vi "seno_gradino.vi"(0 "ampiezza [V]":dbl=10.0, 1 "scelta_funzione":bool, 2 "Gradino_AMP?":bool, 3 "Gradino_FASE?":bool, 5 "frequenza[Hz]":dbl=50.0, 7 "Variazione Percentuale [%]":dbl, 9 "fase[°]":dbl, 11 "Gradi innalzamento[°]":dbl, 12 "rate [sample/s]":dbl=10000.0, 13 "t0[s]":dbl, 14 "lunghezza finestra[s]":dbl=0.06) -> (4 "Waveform Graph":dbl[](graph)=[6.123233995736766e-16, -0.3141075907812828, -0.627905195293134, -0.9410831331851417, -1.2533323356430415, -1.5643446504023082, -1.873813145857246, -2.1814324139654255, -2.4868988716485463, -2.7899110603922934, -3.0901699437494736, -3.3873792024529137, -3.6812455268467796, -3.971478906347807, -4.257792915650727, -4.539904997395467, -4.81753674101715, -5.090414157503713, -5.358267949789969, -5.620833778521307, -5.87785252292473, -6.129070536529766, -6.3742398974868975, -6.613118653236517, -6.845471059286887, -7.071067811865475, -7.289686274214117, -7.501110696304596, -7.705132427757891, -7.901550123756904, -8.090169943749473, -8.270805742745619, -8.443279255020151, -8.607420270039437, -8.763066800438637, -8.910065241883679, -9.048270524660197, -9.177546256839811, -9.297764858882514, -9.408807689542254, -9.510565162951535, -9.60293685676943, -9.685831611286313, -9.759167619387474, -9.822872507286887, -9.876883405951377, -9.921147013144777, -9.9556196460308, -9.980267284282716, -9.995065603657316, -10.0, -9.995065603657316, -9.980267284282716, -9.9556196460308, -9.921147013144779, -9.876883405951379, -9.822872507286887, -9.759167619387474, -9.68583161128631, -9.60293685676943, -9.510565162951536, -9.408807689542254, -9.297764858882513, -9.177546256839811, -9.048270524660195, -8.910065241883677, -8.763066800438635, -8.607420270039437, -8.44327925502015, -8.270805742745619, -8.090169943749476, -7.901550123756903, -7.70513242775789, -7.501110696304597, -7.289686274214116, -7.071067811865474, -6.845471059286886, -6.613118653236519, -6.374239897486895, -6.129070536529765, -5.877852522924733, -5.620833778521309, -5.358267949789964, -5.0904141575037105, -4.817536741017145, -4.539904997395461, -4.257792915650722, -3.971478906347803, -3.6812455268467783, -3.3873792024529137, -3.0901699437494754, -2.789911060392296, -2.486898871648553, -2.1814324139654238, -1.8738131458572462, -1.5643446504023104, -1.2533323356430373, -0.9410831331851397, -0.627905195293132, -0.314107590781283, -1.8369701987210296e-15, 0.3141075907812882, 0.6279051952931372, 0.9410831331851449, 1.2533323356430512, 1.5643446504023157, 1.8738131458572513, 2.181432413965429, 2.4868988716485494, 2.789911060392292, 3.0901699437494723, 3.3873792024529106, 3.6812455268467743, 3.9714789063478073, 4.257792915650726, 4.539904997395467, 4.8175367410171575, 5.090414157503716, 5.358267949789967, 5.620833778521305, 5.877852522924729, 6.1290705365297695, 6.3742398974869, 6.613118653236519, 6.845471059286893, 7.07106781186548, 7.289686274214119, 7.501110696304597, 7.705132427757894, 7.901550123756903, 8.090169943749478, 8.27080574274562, 8.443279255020153, 8.607420270039437, 8.763066800438637, 8.910065241883679, 9.048270524660197, 9.177546256839813, 9.297764858882514, 9.408807689542254, 9.510565162951535, 9.602936856769432, 9.685831611286313, 9.759167619387474, 9.822872507286888, 9.876883405951377, 9.921147013144777, 9.9556196460308, 9.980267284282716, 9.995065603657316, 10.0, 9.995065603657315, 9.980267284282716, 9.9556196460308, 9.921147013144779, 9.876883405951379, 9.822872507286887, 9.759167619387473, 9.68583161128631, 9.60293685676943, 9.510565162951536, 9.408807689542256, 9.297764858882516, 9.177546256839808, 9.048270524660191, 8.910065241883675, 8.763066800438633, 8.607420270039436, 8.443279255020146, 8.270805742745614, 8.09016994374947, 7.901550123756901, 7.70513242775789, 7.501110696304595, 7.28968627421411, 7.071067811865471, 6.845471059286884, 6.613118653236517, 6.374239897486897, 6.129070536529766, 5.8778525229247265, 5.620833778521303, 5.358267949789965, 5.090414157503712, 4.817536741017154, 4.539904997395462, 4.257792915650723, 3.971478906347804, 3.681245526846779, 3.387379202452915, 3.090169943749477, 2.7899110603922885, 2.486898871648546, 2.181432413965425, 1.8738131458572473, 1.5643446504023117, 1.2533323356430472, 0.941083133185132, 0.6279051952931332, 0.31410759078128425, 3.061616997868383e-15, -0.31410759078127803, -0.6279051952931448, -0.9410831331851526, -1.2533323356430501, -1.5643446504023142, -1.8738131458572502, -2.1814324139654278, -2.486898871648548, -2.789911060392308, -3.090169943749471, -3.3873792024529257, -3.681245526846773, -3.9714789063478144, -4.257792915650733, -4.539904997395473, -4.817536741017156, -5.090414157503714, -5.358267949789966, -5.6208337785213045, -5.8778525229247425, -6.129070536529761, -6.3742398974869054, -6.613118653236513, -6.845471059286892, -7.071067811865479, -7.289686274214118, -7.501110696304597, -7.705132427757892, -7.901550123756903, -8.090169943749473, -8.270805742745624, -8.443279255020148, -8.60742027003944, -8.76306680043863, -8.91006524188368, -9.04827052466019, -9.177546256839813, -9.29776485888252, -9.408807689542254, -9.51056516295154, -9.60293685676943, -9.685831611286314, -9.759167619387476, -9.822872507286888, -9.876883405951379, -9.921147013144779, -9.9556196460308, -9.980267284282716, -9.995065603657316, -10.0, -9.995065603657315, -9.980267284282716, -9.955619646030799, -9.921147013144777, -9.876883405951377, -9.822872507286887, -9.759167619387473, -9.68583161128631, -9.602936856769427, -9.510565162951531, -9.40880768954225, -9.29776485888251, -9.177546256839808, -9.048270524660193, -8.910065241883677, -8.763066800438635, -8.607420270039436, -8.443279255020151, -8.270805742745619, -8.090169943749476, -7.901550123756897, -7.705132427757886, -7.50111069630459, -7.289686274214111, -7.071067811865471, -6.845471059286884, -6.613118653236518, -6.3742398974868975, -6.129070536529767, -5.8778525229247345, -5.620833778521311, -5.3582679497899575, -5.090414157503705, -4.817536741017147, -4.539904997395464, -4.2577929156507235, -3.971478906347805, -3.6812455268467636, -3.387379202452916, -3.0901699437494785, -2.7899110603922983, -2.4868988716485556, -2.1814324139654175, -1.8738131458572398, -1.564344650402304, -1.2533323356430395, -0.9410831331851421, -0.6279051952931345, -0.31410759078126765, 1.3477304596986768e-14, 0.31410759078129463, 0.6279051952931436, 0.9410831331851512, 1.2533323356430488, 1.564344650402313, 1.8738131458572491, 2.1814324139654264, 2.486898871648547, 2.78991106039229, 3.09016994374947, 3.387379202452925, 3.6812455268467885, 3.9714789063478135, 4.257792915650732, 4.539904997395472, 4.817536741017155, 5.090414157503713, 5.3582679497899655, 5.620833778521318, 5.877852522924728, 6.129070536529774, 6.374239897486891, 6.6131186532365245, 6.845471059286878, 7.071067811865478, 7.289686274214128, 7.501110696304596, 7.705132427757903, 7.901550123756902, 8.090169943749482, 8.270805742745624, 8.443279255020157, 8.607420270039439, 8.76306680043864, 8.91006524188368, 9.048270524660204, 9.177546256839811, 9.29776485888252, 9.408807689542254, 9.51056516295154, 9.602936856769428, 9.685831611286313, 9.759167619387476, 9.822872507286888, 9.876883405951379, 9.921147013144779, 9.9556196460308, 9.980267284282716, 9.995065603657316, 10.0, 9.995065603657316, 9.980267284282716, 9.9556196460308, 9.921147013144777, 9.876883405951377, 9.822872507286887, 9.759167619387474, 9.685831611286313, 9.602936856769432, 9.510565162951533, 9.408807689542257, 9.29776485888251, 9.177546256839817, 9.048270524660193, 8.910065241883668, 8.763066800438635, 8.607420270039427, 8.443279255020151, 8.27080574274561, 8.090169943749467, 7.9015501237568975, 7.705132427757887, 7.501110696304591, 7.289686274214111, 7.071067811865472, 6.845471059286885, 6.613118653236505, 6.374239897486898, 6.1290705365297535, 5.877852522924735, 5.6208337785212965, 5.358267949789958, 5.090414157503707, 4.817536741017149, 4.539904997395465, 4.257792915650725, 3.97147890634779, 3.6812455268467814, 3.3873792024529004, 3.0901699437494794, 2.7899110603922823, 2.4868988716485565, 2.181432413965419, 1.8738131458572238, 1.5643446504023053, 1.2533323356430408, 0.9410831331851434, 0.6279051952931357, 0.31410759078126893, 5.5109105961630896e-15, -0.3141075907812934, -0.6279051952931247, -0.94108313318515, -1.253332335643065, -1.564344650402312, -1.873813145857265, -2.1814324139654255, -2.486898871648563, -2.789911060392289, -3.0901699437494856, -3.387379202452924, -3.6812455268467876, -3.971478906347812, -4.257792915650731, -4.539904997395471, -4.817536741017169, -5.090414157503713, -5.35826794978998, -5.620833778521303, -5.877852522924742, -6.129070536529772, -6.374239897486904, -6.613118653236524, -6.845471059286891, -7.071067811865478, -7.289686274214117, -7.501110696304595, -7.705132427757903, -7.901550123756901, -8.090169943749482, -8.270805742745614, -8.443279255020155, -8.607420270039448, -8.763066800438638, -8.910065241883688, -9.048270524660197, -9.177546256839818, -9.297764858882513, -9.40880768954226, -9.51056516295154, -9.602936856769434, -9.685831611286313, -9.75916761938747, -9.822872507286887, -9.87688340595138, -9.921147013144779, -9.955619646030803, -9.980267284282716, -9.995065603657316, -10.0, -9.995065603657315, -9.980267284282716, -9.9556196460308, -9.921147013144777, -9.876883405951377, -9.822872507286887, -9.759167619387469, -9.685831611286313, -9.602936856769427, -9.510565162951544, -9.408807689542257, -9.29776485888251, -9.1775462568398, -9.048270524660193, -8.910065241883686, -8.763066800438637, -8.607420270039427, -8.443279255020151, -8.27080574274561, -8.090169943749478, -7.9015501237568975, -7.705132427757899, -7.5011106963045915, -7.2896862742141, -7.071067811865474, -6.845471059286873, -6.613118653236519, -6.374239897486885, -6.129070536529769, -5.877852522924723, -5.620833778521284, -5.35826794978996, -5.090414157503723, -4.8175367410171495, -4.539904997395451, -4.257792915650694, -3.9714789063478233, -3.6812455268467827, -3.3873792024529017, -3.090169943749447, -2.789911060392283, -2.486898871648558, -2.1814324139654198, -1.873813145857225, -1.5643446504023064, -1.2533323356430246, -0.9410831331851445, -0.6279051952931192, -0.3141075907812879, 1.1028010998692062e-14, 0.31410759078127437, 0.6279051952931413, 0.9410831331851666, 1.2533323356430461, 1.564344650402293, 1.8738131458572465, 2.1814324139654415, 2.486898871648579, 2.7899110603922708, 3.090169943749468, 3.3873792024529226, 3.681245526846803, 3.971478906347844, 4.257792915650714, 4.539904997395469, 4.817536741017168, 5.0904141575037425, 5.358267949790009, 5.620833778521302, 5.877852522924741, 6.129070536529786, 6.374239897486929, 6.613118653236509, 6.84547105928689, 7.071067811865489, 7.28968627421414, 7.501110696304583, 7.70513242775789, 7.901550123756911, 8.09016994374949, 8.270805742745603, 8.443279255020146, 8.607420270039439, 8.763066800438645, 8.910065241883697, 9.048270524660188, 9.177546256839811, 9.29776485888252, 9.408807689542265, 9.510565162951528, 9.602936856769428, 9.685831611286313, 9.75916761938748, 9.822872507286894, 9.876883405951375, 9.921147013144779, 9.9556196460308, 9.980267284282718, 9.995065603657316, 10.0, 9.995065603657315, 9.980267284282714, 9.955619646030797, 9.921147013144779, 9.876883405951377, 9.822872507286885, 9.759167619387467, 9.685831611286316, 9.602936856769432, 9.510565162951533, 9.408807689542245, 9.297764858882525, 9.177546256839817, 9.048270524660193, 8.91006524188367, 8.763066800438619, 8.607420270039446, 8.443279255020153, 8.270805742745612, 8.090169943749459, 7.901550123756876, 7.705132427757899, 7.501110696304592, 7.289686274214101, 7.071067811865449, 6.845471059286848, 6.613118653236521, 6.374239897486886, 6.129070536529742, 5.877852522924751, 5.620833778521313, 5.358267949789961, 5.090414157503693, 4.817536741017181, 4.5399049973954835, 4.257792915650727, 3.971478906347792, 3.6812455268467503, 3.3873792024529363, 3.0901699437494816, 2.789911060392285, 2.4868988716485245, 2.1814324139653865, 1.873813145857261, 1.5643446504023077, 1.2533323356430257, 0.9410831331851104, 0.6279051952930849, 0.3141075907812891], 6 "Ampiezza":dbl[](array[numeric]), 10 "Fase":dbl[](array[numeric]), 15 "Frequenza":dbl[](array[numeric]))   [LabVIEW 2019]
doc: "questo VI calcola un seno o un coseno"
panel:
  out "Grafico":cluster{dbl, dbl, dbl[]}(graph)
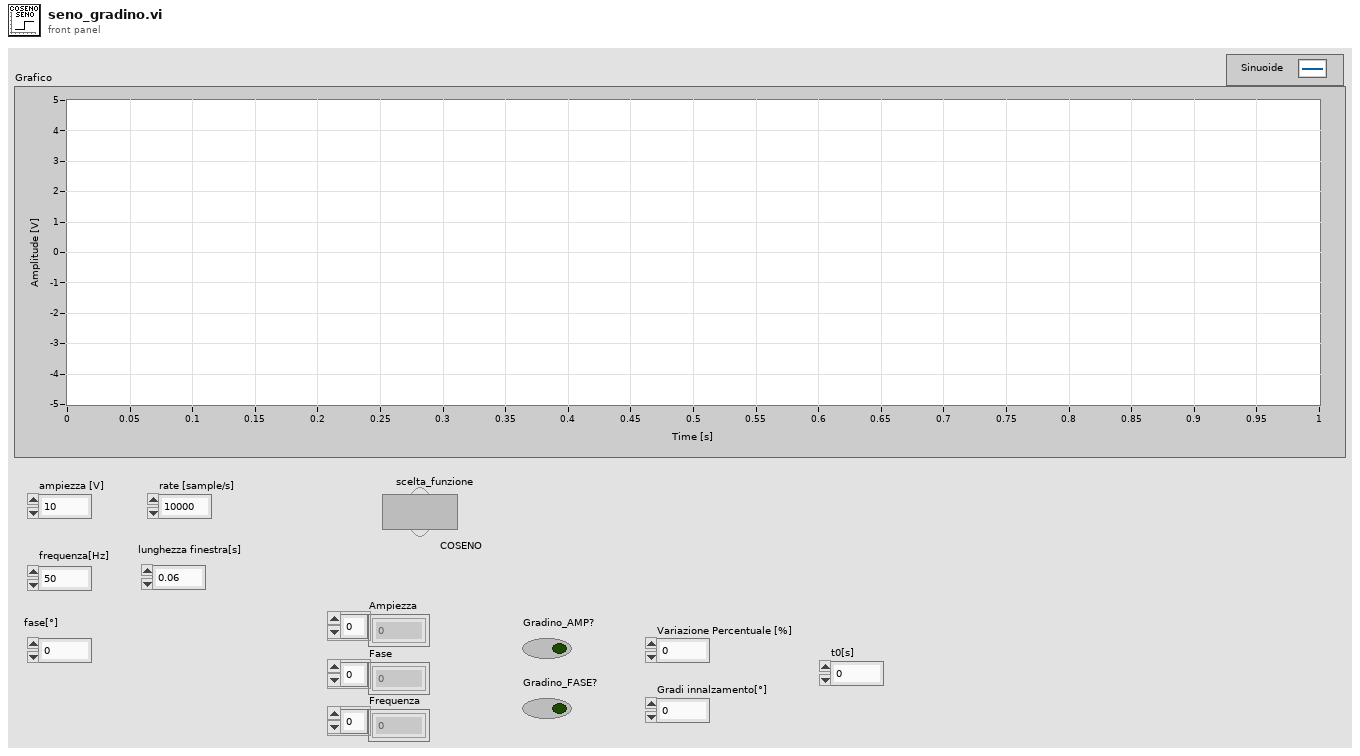
[diagram p1: front panel]
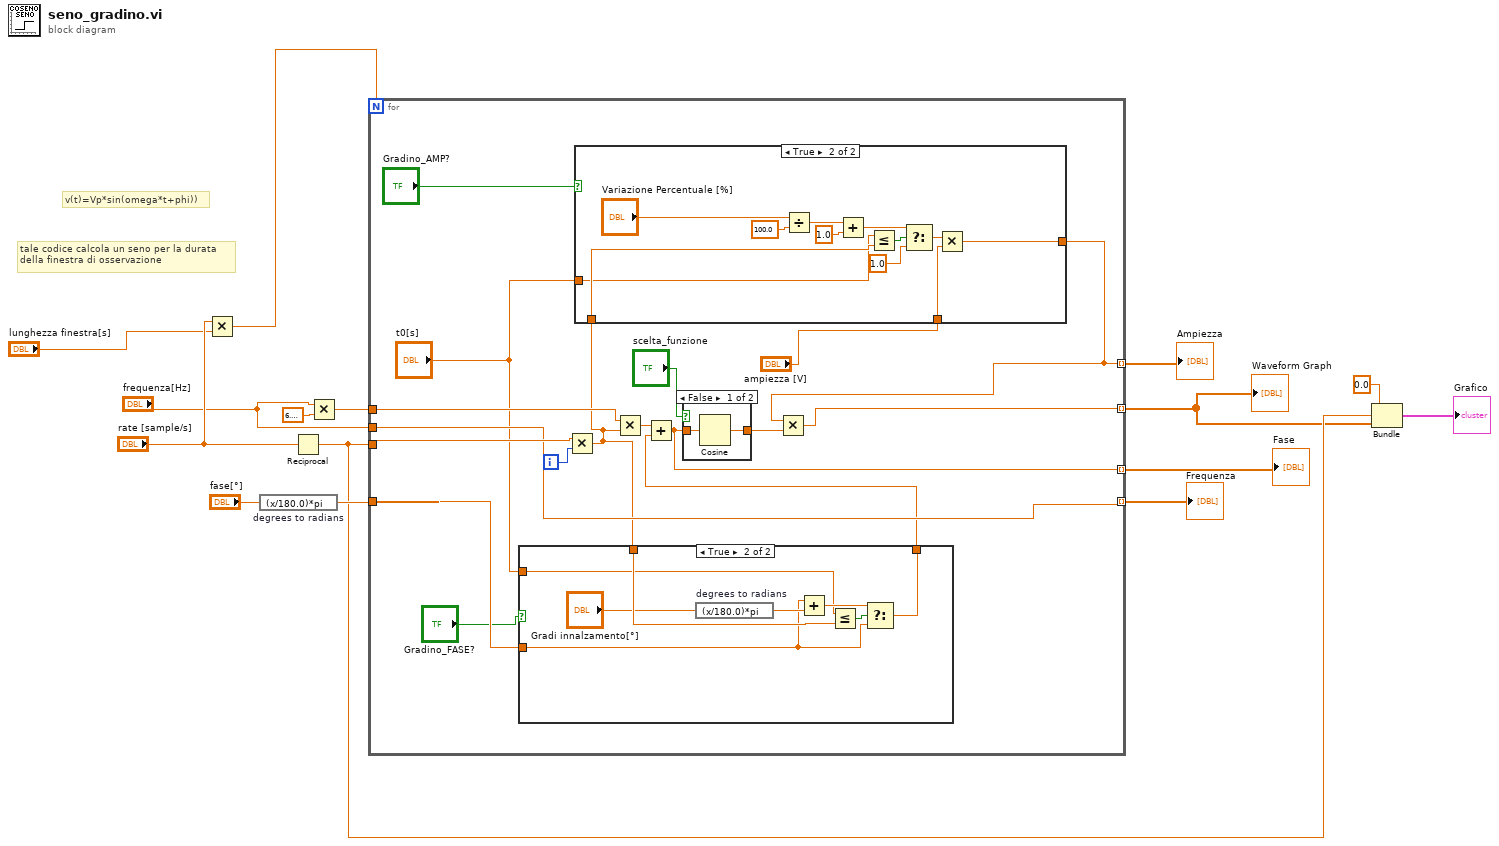
[diagram p0: block diagram]
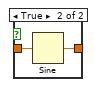
[diagram p4: hidden frame]
diagram:
  # "v(t)=Vp*sin(omega*t+phi))"
  # "tale codice calcola un seno per la durata \ndella finestra di osservazione"
  n1 = Multiply(x="rate [sample/s]", y="lunghezza finestra[s]") -> (x*y=w15:dbl)
  n2 = expression code="(x/180.0)*pi" "degrees to radians"("fase[°]") -> (w10:dbl)
  n3 = Reciprocal(x="rate [sample/s]") -> (1/x=w8:dbl)
  n4 = Multiply(x="frequenza[Hz]", y=6.283185307179586) -> (x*y=w12:dbl)
  n5 = for {
    N: w15 -> [_]
    tunnel: w8 -> [w31]
    tunnel: w12 -> [w30]
    tunnel: w10 -> [w19]
    tunnel: [w27] -> w7 mode=indexing
    tunnel: [w23] -> w5 mode=indexing
    tunnel: [w25] -> w4 mode=indexing
    tunnel: "frequenza[Hz]" -> [w24]
    tunnel: [w24] -> w2 mode=indexing
    i -> [w32]
    n6 = Multiply(x=w31, y=w32) -> (x*y=w20:dbl)
    n7 = case shown="True" "Gradino_FASE?" {
      tunnel: w20 -> [_ w41]
      tunnel: w19 -> [w33 w36]
      tunnel: [w33 w35] -> w18
      tunnel: "t0[s]" -> [_ w34]
      frame False {
      }
      frame True {
        n8 = expression code="(x/180.0)*pi" "degrees to radians"("Gradi innalzamento[°]") -> (w39:dbl)
        n9 = Add(x=w36, y=w39) -> (x+y=w38:dbl)
        n10 = Less Or Equal?(x=w34, y=w41) -> (x <= y?=w37:bool)
        n11 = Select(t=w38, s=w37, f=w36) -> (s? t:f=w35:dbl)
      }
    }
    n12 = case shown="True" "Gradino_AMP?" {
      tunnel: w20 -> [_ w54]
      tunnel: [w42 w45] -> w23
      tunnel: "ampiezza [V]" -> [w42 w44]
      tunnel: "t0[s]" -> [_ w43]
      frame False {
      }
      frame True {
        n13 = Divide(x="Variazione Percentuale [%]", y=100.0) -> (x/y=w51:dbl)
        n14 = Add(x=w51, y=1.0) -> (x+y=w50:dbl)
        n15 = Less Or Equal?(x=w43, y=w54) -> (x <= y?=w49:bool)
        n16 = Select(t=w50, s=w49, f=1.0) -> (s? t:f=w48:dbl)
        n17 = Multiply(x=w48, y=w44) -> (x*y=w45:dbl)
      }
    }
    n18 = Multiply(x=w30, y=w20) -> (x*y=w29:dbl)
    n19 = Add(x=w29, y=w18) -> (x+y=w25:dbl)
    n20 = case shown="False" "scelta_funzione" {
      tunnel: w25 -> [w56 w58]
      tunnel: [w55 w57] -> w28
      frame False {
        n21 = Cosine(x=w56) -> (cos(x)=w55:dbl)
      }
      frame True {
        n22 = Sine(x=w58) -> (sin(x)=w57:dbl)
      }
    }
    n23 = Multiply(x=w23, y=w28) -> (x*y=w27:dbl)
  }
  "Waveform Graph" <- w7
  "Ampiezza" <- w5
  "Fase" <- w4
  "Frequenza" <- w2
  n24 = Bundle(0.0, w8, w7) -> (→"Grafico":cluster{dbl, dbl, dbl[]})  [unwired: 1 in]
